vi "9700 Invalid Enqueuer Ident--error.vi"(8 "error in":errorcluster, 11 "Ident":string) -> (0 "error out":errorcluster)   [LabVIEW 2024, in "Network Management UI.lvlib" / "Network Management UI.lvclass"]
uses:
  Network Management UI.lvclass
  Network Management UI.lvclass/Network Management UI.ctl
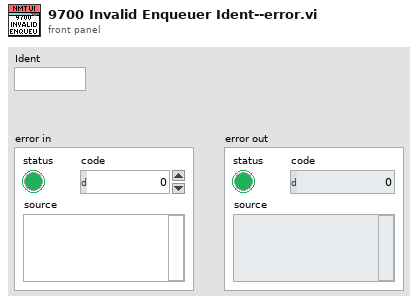
[diagram p1: front panel]
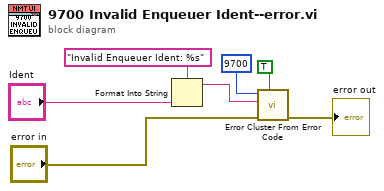
[diagram p0: block diagram]
diagram:
  n1 = Format Into String(format string="Invalid Enqueuer Ident: %s" ("error message (\"\")"), "Ident") -> (resulting string=w5:string)  [unwired: 2 in, 1 out]
  n2 = call <vilib>:"Error Cluster From Error Code.vi"("show call chain? (False)"=TRUE, "error in (no error)"="error in", "error message (\"\")"=w5, "error code (0)"=9700) -> ("error out"=→"error out":errorcluster)  [unwired: 5 in]
